vi "To VConfig.vi"(8 "error in (no error)":errorcluster, 11 "Modbus TCP Micro Master in":refnum<class "Modbus TCP Micro Master.lvclass">) -> (0 "error out":errorcluster, 2 "variant":variant, 3 "Modbus TCP Micro Master out":refnum<class "Modbus TCP Micro Master.lvclass">)   [LabVIEW 2023, in "Modbus TCP Micro.lvlib" / "Modbus TCP Micro Master.lvclass"]
uses:
  Modbus TCP Micro Master.lvclass
  Modbus TCP Micro Master.lvclass/Modbus TCP Micro Master.ctl
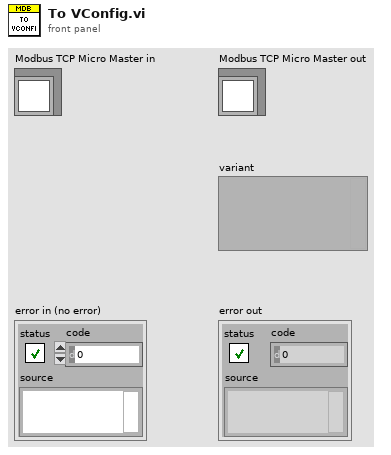
[diagram p1: front panel]
types:
  T1 = typedef "Modbus TCP Micro.lvlib/Modbus TCP Micro Master.lvclass/Settings.ctl" = cluster{"address":string, "remote port or service name":u16, "timeout ms (10000)":i32, "local port (0)":u16}
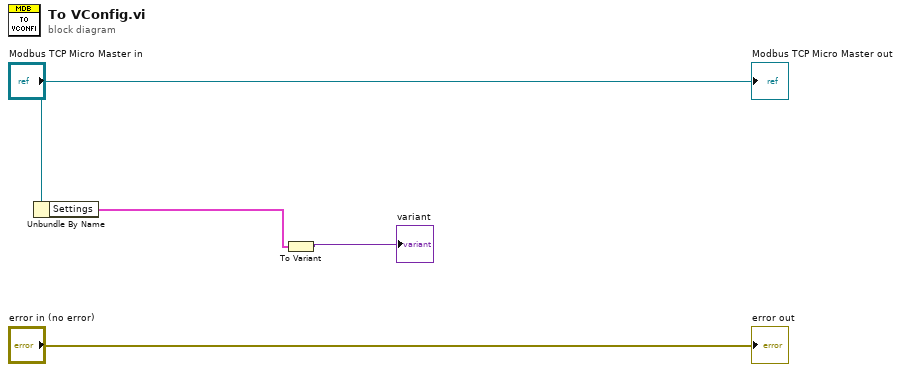
[diagram p0: block diagram]
diagram:
  n1 = Unbundle By Name("Modbus TCP Micro Master in") -> ("Settings"=w2:T1)
  n2 = To Variant(anything=w2) -> (Variant=→"variant":variant)
  "error out" <- "error in (no error)"
  "Modbus TCP Micro Master out" <- "Modbus TCP Micro Master in"
